vi "Graphs.vi"(8 "error in (no error)":errorcluster, 9 "Clear Graphs":bool, 11 "Position":dbl[](array[numeric])) -> (0 "error out":errorcluster)   [LabVIEW 2018, in "Stage Actor.lvlib" / "Stage.lvclass"]
uses:
  Stage.lvclass
  <vilib>/Native 3D Graph/xcontrol/3DPC_SurfacePlot.xctl
  <vilib>/MGI/Panel Manager/Panel/Panel/Window/Window.lvclass
  C:/Program Files/National Instruments/LabVIEW 2018/vi.lib/MGI/Panel Manager/Panel/Panel/Panel.lvclass
  <vilib>/MGI/Panel Manager/Panel/Panel/Window/Window.vi
  <vilib>/MGI/Panel Manager/Panel/Panel/Panel.lvclass
  <vilib>/MGI/Panel Manager/Panel/Panel.lvlib
  ADM/Main.lvlib
panel:
  in  "New Layer":bool
  out "YZ Graph":cluster{"Y":dbl[], "Z":dbl[]}(graph)
  out "XY Graph":cluster{"X":dbl[], "Y":dbl[]}(graph)
  out "3D Graph":refnum<class "Base Datatype.lvclass">[](xcontrol)
  out "XZ Graph":cluster{"X":dbl[], "Z":dbl[]}(graph)
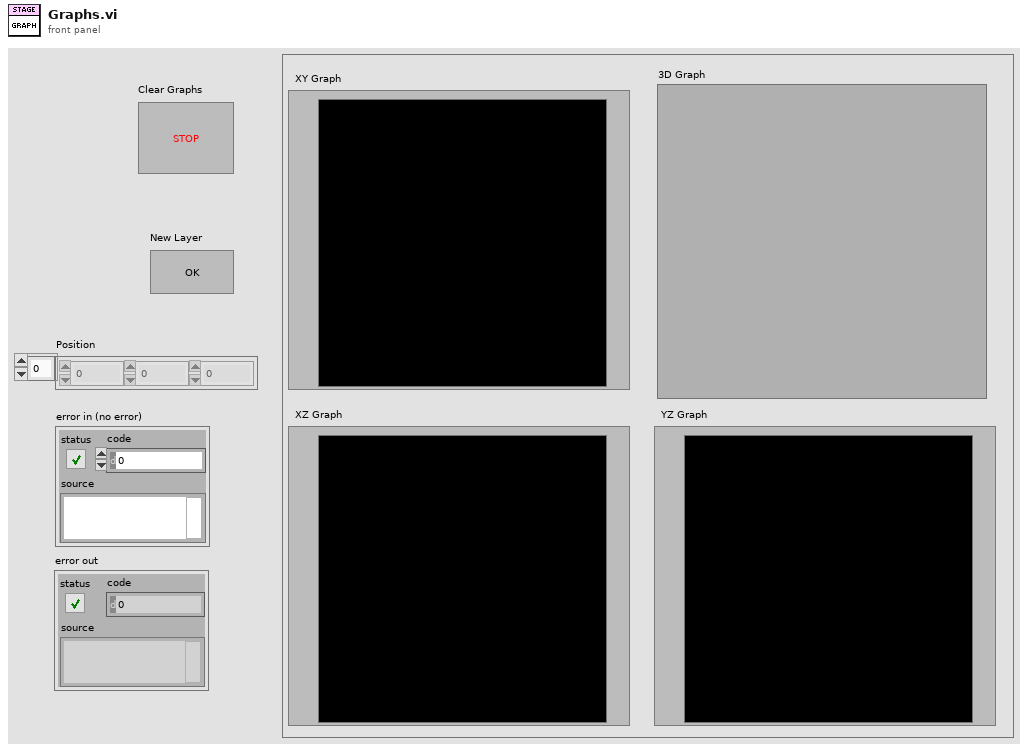
[diagram p1: front panel]
types:
  T1 = cluster{"Position[0]":dbl, "Position[1]":dbl, "Position[2]":dbl, "Position[3]":dbl, "Position[4]":dbl, "Position[5]":dbl, "Position[6]":dbl, "Position[7]":dbl, "Position[8]":dbl}
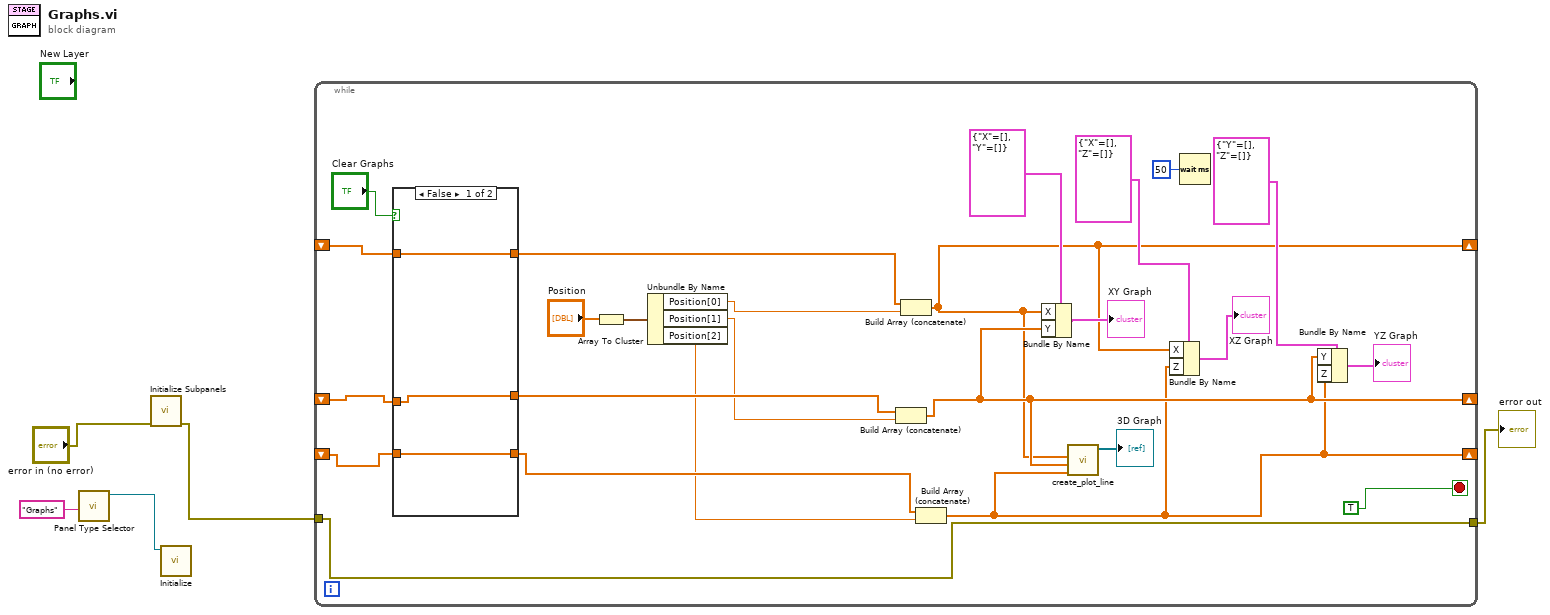
[diagram p0: block diagram]
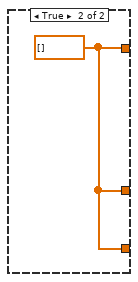
[diagram p2: hidden frame]
diagram:
  n1 = call-poly <vilib>:"Panel Type Selector.vi"("Default Title"="Graphs") -> ("Window out"=w5:refnum<class "Window.lvclass">)  [unwired: 9 in, 1 out]
  n2 = call "Initialize Subpanels.vi"("error in (no error)"="error in (no error)") -> ("error out"=w2:errorcluster)  [unwired: 10 in]
  n3 = call <vilib>:"Initialize.vi"("Panel In"=w5) -> ()  [unwired: 8 in, 3 out]
  n4 = while {
    shift-right: [w21] -> _
    shift-left: _ -> [w16]
    shift-right: [w23] -> _
    shift-left: _ -> [w14]
    shift-right: [w20] -> _
    shift-left: _ -> [w12]
    tunnel: w2 -> [w18]
    tunnel: [w18] -> w1
    stop <- TRUE stop-if-true
    n5 = case shown="False" "Clear Graphs" {
      tunnel: w16 -> [w33 _]
      tunnel: [w33 w34] -> w15
      tunnel: w14 -> [w32 _]
      tunnel: [w32 w34] -> w13
      tunnel: [w31 w34] -> w11
      tunnel: w12 -> [w31 _]
      frame False {
      }
      frame True {
        w34 = dbl[] []
      }
    }
    n6 = Array To Cluster(array="Position") -> (cluster=w10:T1)
    n7 = Unbundle By Name(w10) -> ("Position[0]"=w8:dbl, "Position[1]"=w7:dbl, "Position[2]"=w6:dbl)
    n8 = Build Array (concatenate)(w13, w7) -> (w23:dbl[])
    n9 = Build Array (concatenate)(w15, w8) -> (w21:dbl[])
    n10 = Build Array (concatenate)(w11, w6) -> (w20:dbl[])
    n11 = Bundle By Name(cluster=cluster{"X":dbl[], "Y":dbl[]} {"X"=[], "Y"=[]} ("Cluster"), "X"=w21, "Y"=w23) -> (→"XY Graph":cluster{"X":dbl[], "Y":dbl[]})
    n12 = call <vilib>:"create_plot_line.vi"("z vector"=w20, "y vector"=w23, "x vector"=w21) -> ("plots out"=→"3D Graph":refnum<class "Base Datatype.lvclass">[])  [unwired: 2 in, 6 out]
    n13 = Bundle By Name(cluster=cluster{"X":dbl[], "Z":dbl[]} {"X"=[], "Z"=[]} ("Cluster"), "X"=w21, "Z"=w20) -> (→"XZ Graph":cluster{"X":dbl[], "Z":dbl[]})
    n14 = Wait (ms)(milliseconds to wait=u32 50) -> ()  [unwired: 1 out]
    n15 = Bundle By Name(cluster=cluster{"Y":dbl[], "Z":dbl[]} {"Y"=[], "Z"=[]} ("Cluster"), "Y"=w23, "Z"=w20) -> (→"YZ Graph":cluster{"Y":dbl[], "Z":dbl[]})
  }
  "error out" <- w1
